vi "AlliGator Load Extended PTU File Information.vi"(8 "Error In":errorcluster, 11 "File Path":path) -> (0 "Error Out":errorcluster, 1 "Data Description":string, 2 "Version":string, 3 "FLI Data File Information":T15, 4 "Load Time (s)":dbl, 5 "Extended ptu File Information":T1, 6 "Magic":string)   [LabVIEW 2021, in "AlliGator Files.lvlib"]
doc: "Extracts metadata used to load FLI dataset from .ptu file."
uses:
  AlliGator Files.lvlib
  AlliGator FLI Data File Information.ctl
  Phasor/Phasor Fluorescence Lifetime Parameters v3.ctl
  AlliGator FLI Dataset Type.ctl
  PicoQuant/PTU/LabVIEW/Extended PicoQuant Data File Information.ctl
  PicoQuant/PTU/LabVIEW/PicoQuant Data File Information.ctl
  PicoQuant/PTU/LabVIEW/PicoQuant File Information.ctl
  PicoQuant/PTU/LabVIEW/PicoQuant Software Information.ctl
  PicoQuant/PTU/LabVIEW/PicoQuant Remote Request Information.ctl
  PicoQuant/PTU/LabVIEW/PicoQuant Hardware Information.ctl
  PicoQuant/PTU/LabVIEW/PicoQuant Input Channels.ctl
  PicoQuant/PTU/LabVIEW/PicoQuant Markers.ctl
  PicoQuant/PTU/LabVIEW/PicoQuant Modules.ctl
  PicoQuant/PTU/LabVIEW/PicoQuant Router Channels.ctl
  PicoQuant/PTU/LabVIEW/PicoQuant Measurement Information.ctl
  PicoQuant/PTU/LabVIEW/PicoQuant Image Information.ctl
  PicoQuant/PTU/LabVIEW/PicoQuant Results Format.ctl
  PicoQuant/PTU/LabVIEW/PicoQuant Measurement Results.ctl
  AlliGator Settings List.ctl
  Variant/Variant to Data/Variant to U32.vi
  AlliGator Load Single Gate Image from PTU File.vi
  PicoQuant/PTU/LabVIEW/PTU Files.lvlib
  PicoQuant/PicoQuant.lvlib
  AlliGator HDF5.lvlib
  AlliGator Settings.lvlib
  Variant/Variant to Data/Variant to Data.lvlib
  Phasor/Phasor.lvlib
panel:
  # "see the AlliGator License on the block diagram (Ctrl+E or Window:Show Block Diagram)"
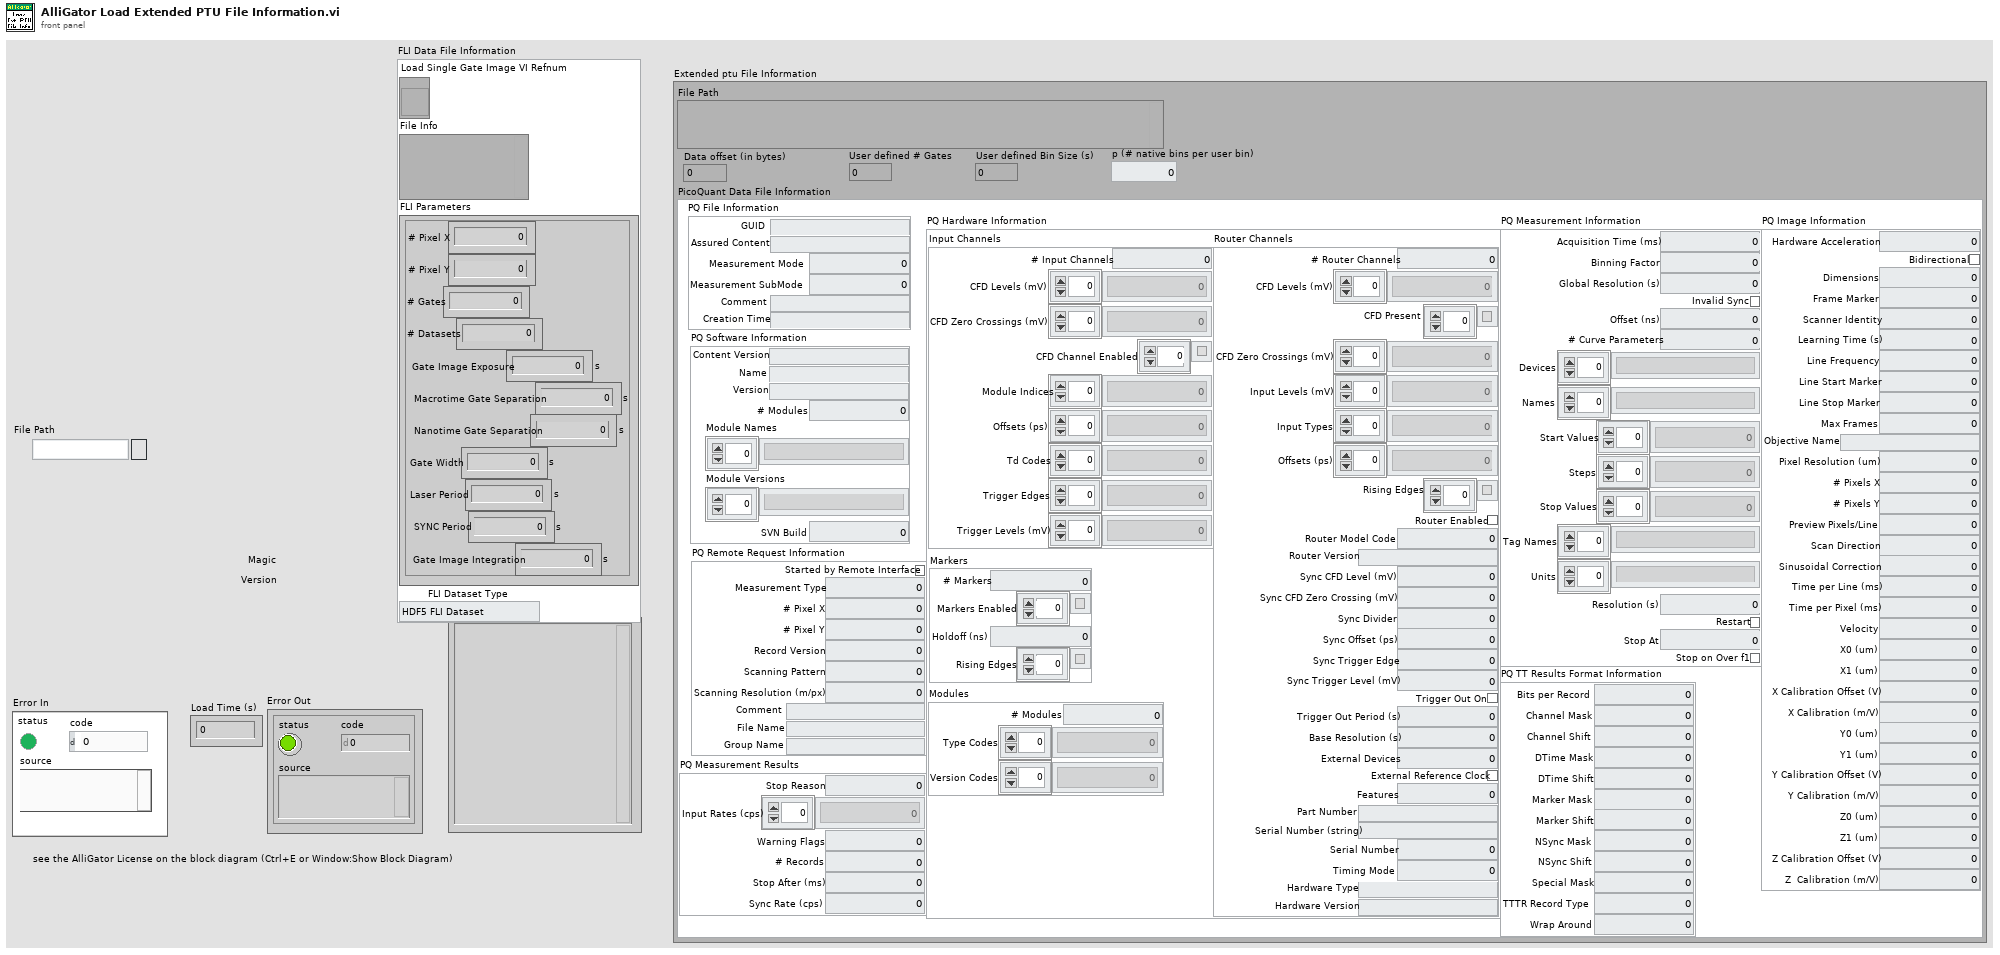
[diagram p1: front panel]
types:
  T1 = typedef "PicoQuant.lvlib/Extended PicoQuant Data File Information.ctl" = cluster{"File Path":path, "Data offset (in bytes)":i64, "PicoQuant Data File Information":T2, "User defined # Gates":i64, "User defined Bin Size (s)":dbl, "p (# native bins per user bin)":dbl}
  T2 = typedef "PTU Files.lvlib/PicoQuant Data File Information.ctl" = cluster{"PQ File Information":T3, "PQ Software Information":T4, "PQ Remote Request Information":T5, "PQ Hardware Information":T6, "PQ Measurement Information":T11, "PQ Image Information":T12, "PQ TT Results Format Information":T13, "PQ Measurement Results":T14}
  T3 = typedef "PTU Files.lvlib/PicoQuant File Information.ctl" = cluster{"GUID":string, "Assured Content":string, "Measurement Mode":i64, "Measurement SubMode":i64, "Comment":string, "Creation Time":string}
  T4 = typedef "PTU Files.lvlib/PicoQuant Software Information.ctl" = cluster{"Content Version":string, "Name":string, "Version":string, "# Modules":i64, "Module Names":string[], "Module Versions":string[], "SVN Build":i64}
  T5 = typedef "PTU Files.lvlib/PicoQuant Remote Request Information.ctl" = cluster{"Started by Remote Interface":bool, "Measurement Type":i64, "# Pixel X":i64, "# Pixel Y":i64, "Record Version":i64, "Scanning Pattern":i64, "Scanning Resolution (m/px)":dbl, "Comment":string, "File Name":string, "Group Name":string}
  T6 = typedef "PTU Files.lvlib/PicoQuant Hardware Information.ctl" = cluster{"Input Channels":T7, "Markers":T8, "Modules":T9, "Router Channels":T10}
  T7 = typedef "PTU Files.lvlib/PicoQuant Input Channels.ctl" = cluster{"# Input Channels":i64, "CFD Levels (mV)":i64[], "CFD Zero Crossings (mV)":i64[], "CFD Channel Enabled":bool[], "Module Indices":i64[], "Offsets (ps)":i64[], "Td Codes":i64[], "Trigger Edges":i64[], "Trigger Levels (mV)":i64[]}
  T8 = typedef "PTU Files.lvlib/PicoQuant Markers.ctl" = cluster{"# Markers":i64, "Markers Enabled":bool[], "Holdoff (ns)":i64, "Rising Edges":bool[]}
  T9 = typedef "PTU Files.lvlib/PicoQuant Modules.ctl" = cluster{"# Modules":i64, "Type Codes":i64[], "Version Codes":i64[]}
  T10 = typedef "PTU Files.lvlib/PicoQuant Router Channels.ctl" = cluster{"# Router Channels":i64, "CFD Levels (mV)":i64[], "CFD Present":bool[], "CFD Zero Crossings (mV)":i64[], "Input Levels (mV)":i64[], "Input Types":i64[], "Offsets (ps)":i64[], "Rising Edges":bool[], "Router Enabled":bool, "Router Model Code":i64, "Router Version":string, "Sync CFD Level (mV)":i64, "Sync CFD Zero Crossing (mV)":i64, "Sync Divider":i64, "Sync Offset (ps)":i64, "Sync Trigger Edge":i64, "Sync Trigger Level (mV)":i64, "Trigger Out On":bool, "Trigger Out Period (s)":dbl, "Base Resolution (s)":dbl, "External Devices":i64, "External Reference Clock":bool, "Features":u64, "Part Number":string, "Serial Number (string)":string, "Serial Number":i64, "Timing Mode":i64, "Hardware Type":string, "Hardware Version":string}
  T11 = typedef "PTU Files.lvlib/PicoQuant Measurement Information.ctl" = cluster{"Acquisition Time (ms)":i64, "Binning Factor":i64, "Global Resolution (s)":dbl, "Invalid Sync":bool, "Offset (ns)":u64, "# Curve Parameters":u64, "Devices":string[], "Names":string[], "Start Values":dbl[], "Steps":dbl[], "Stop Values":dbl[], "Tag Names":string[], "Units":string[], "Resolution (s)":dbl, "Restart":bool, "Stop At":u64, "Stop on Over f1":bool}
  T12 = typedef "PTU Files.lvlib/PicoQuant Image Information.ctl" = cluster{"Hardware Acceleration":i64, "Bidirectional":bool, "Dimensions":i64, "Frame Marker":i64, "Scanner Identity":i64, "Learning Time (s)":i64, "Line Frequency":dbl, "Line Start Marker":i64, "Line Stop Marker":i64, "Max Frames":i64, "Objective Name":string, "Pixel Resolution (um)":dbl, "# Pixels X":i64, "# Pixels Y":i64, "Preview Pixels/Line":i64, "Scan Direction":i64, "Sinusoidal Correction":i64, "Time per Line (ms)":dbl, "Time per Pixel (ms)":i64, "Velocity":i64, "X0 (um)":dbl, "X1 (um)":dbl, "X Calibration Offset (V)":dbl, "X Calibration (m/V)":dbl, "Y0 (um)":dbl, "Y1 (um)":dbl, "Y Calibration Offset (V)":dbl, "Y Calibration (m/V)":dbl, "Z0 (um)":dbl, "Z1 (um)":dbl, "Z Calibration Offset (V)":dbl, "Z  Calibration (m/V)":dbl}
  T13 = typedef "PTU Files.lvlib/PicoQuant Results Format.ctl" = cluster{"Bits per Record":i64, "Channel Mask":i64, "Channel Shift ":i64, "DTime Mask":i64, "DTime Shift":i64, "Marker Mask":i64, "Marker Shift":i64, "NSync Mask":i64, "NSync Shift":i64, "Special Mask":i64, "TTTR Record Type":i64, "Wrap Around":i64}
  T14 = typedef "PTU Files.lvlib/PicoQuant Measurement Results.ctl" = cluster{"Stop Reason":i64, "Input Rates (cps)":i64[], "Warning Flags":u64, "# Records":i64, "Stop After (ms)":i64, "Sync Rate (cps)":i64}
  T15 = typedef "AlliGator HDF5.lvlib/AlliGator FLI Data File Information.ctl" = cluster{"Load Single Gate Image VI Refnum":refnum<vi>, "File Info":variant, "FLI Parameters":T16, "FLI Dataset Type":T17}
  T16 = typedef "Phasor.lvlib/Phasor Fluorescence Lifetime Parameters v3.ctl" = cluster{"# Pixel X":i32, "# Pixel Y":i32, "# Gates":i32, "# Datasets":i32, "Gate Image Exposure":dbl[unit], "Macrotime Gate Separation":dbl[unit], "Nanotime Gate Separation":dbl[unit], "Gate Width":dbl[unit], "Laser Period":dbl[unit], "SYNC Period":dbl[unit], "Gate Image Integration":dbl[unit]}
  T17 = typedef "AlliGator Files.lvlib/AlliGator FLI Dataset Type.ctl" = enum16{"HDF5 FLI Dataset", "Gate Image Folder", ".sdt FLI Dataset (Becker & Hickl)", ".ptu FLI Dataset (PicoQuant)", "SS1 FLI Dataset", "SS2 FLI Dataset", "I/m/phi Dataset", ".bin FLI Dataset (PicoQuant Binned)", ".bin FLI Dataset (Piccolo Binned)"}
  T18 = typedef "AlliGator Settings.lvlib/AlliGator Settings List.ctl" = enum16{"GUI:Visible Settings Tab", "GUI:Last Run Version", "Source Image:Use Image Histogram for Contrast", "Source Image:Low Count Pixels Rejection Options", "Source Image:High Count Pixels Rejection Options", "Source Image:Use Image Brightness", "Source Image:Blend Overlay with Image Background", "Source Image:Use Fixed ROI Diameter", "Source Image:ROI Diameter", "Source Image:ROI Center Color", "Source Image:Peak Threshold", "Source Image:Intensity Threshold", "Source Image:Image Binning Options", "Source Image:Image Smoothing Options", "Source Image:Image Histogram Active", "Source Image:Invert Binary Mask", "Source Image:Hot Pixel Removal", "Source Image:Overlay Analyzed ROI Center", "Source Image:Auto-Adjust Contrast", "Source Image:Histogram Lower Percentile", "Source Image:Histogram Upper Percentile", "Source Image:Save Source Image", "Source Image:Scale Bar Options", "Source Image:Image Resolution (Pixel Size)", "Source Image:Flatfield Correction", "Source Image:Show Dead Left Columns Correction", "Source Image:Dead Left Columns Correction", "Source Image:Image Pre-Processing Operations Order", "Source Image:Overlay ROI Median", "Source Image:Median Overlay Color", "Data Information:Gate Width", "Data Information:Nanotime Gate Separation", "Data Information:Macrotime Gate Separation", "Data Information:Gate Step", "Data Information:# Gates", "Data Information:Gate Image Exposure", "Data Information:Gate Image Integration", "Data Information:Gates to Skip", "Data Information:Gates to Keep", "Data Information:Define Gates to", "Data Information:Channel Name", "Data Information:Available Channel Names", "Data Information:Channel Arithmetic", "Data Information:Background File Subtraction", "Data Information:Background File", "Data Information:Background Scaling Factor", "Data Information:Background Pile-up Correction", "Data Information:Background Pixel Well Capacity", "Data Information:Laser Period", "Data Information:SYNC Period", "Data Information:Pile-up Correction", "Data Information:Pixel Well Capacity", "Data Information:Dataset Scaling Factor", "Fluorescence Decay_Decay Pre-Processing:Reverse Gates", "Fluorescence Decay_Decay Pre-Processing:Verbose Decay Pre-Processing", "Fluorescence Decay_Decay Pre-Processing:Use Decay Pre-Processing", "Fluorescence Decay_Decay Pre-Processing:Background Subtraction", "Fluorescence Decay_Decay Pre-Processing:Background Definition Range", "Fluorescence Decay_Decay Pre-Processing:Baseline Subtraction Method", "Fluorescence Decay_Decay Pre-Processing:Decay Pre-Processing Operations Order", "Fluorescence Decay_Decay Pre-Processing:Smoothing Parameter", "Fluorescence Decay_Decay Pre-Processing:Shift Decay", "Fluorescence Decay_Decay Pre-Processing:Decay Shift Parameters", "Fluorescence Decay_Decay Pre-Processing:Fold Decay", "Fluorescence Decay_Decay Pre-Processing:# Folds", "Fluorescence Decay_Decay Pre-Processing:1-Normalize Decay", "Fluorescence Decay_Decay Pre-Processing:[0-1]-Normalize Decay", "Fluorescence Decay_Decay Pre-Processing:Smoothen Decay", "Fluorescence Decay_Decay Pre-Processing:Extrapolate Decay", "Fluorescence Decay_Decay Pre-Processing:Use Periodicity", "Fluorescence Decay_Decay Pre-Processing:Use Cursors", "Fluorescence Decay_Decay Pre-Processing:Tail Fraction", "Fluorescence Decay_Decay Pre-Processing:Head Fraction", "Fluorescence Decay_Decay Pre-Processing:Additional Points", "Fluorescence Decay_Decay Pre-Processing:Straighten Decay", "Fluorescence Decay_Decay Pre-Processing:Constant Background", "Fluorescence Decay_Decay Pre-Processing:Pixel-Normalize Decay", "Fluorescence Decay_Advanced Analysis:Extract IRF instead of Decay", "Fluorescence Decay_Advanced Analysis:IRF Extraction Options", "Fluorescence Decay_Advanced Analysis:IRF Optimization Options", "Fluorescence Decay_Advanced Analysis:Square Pulse Options", "Fluorescence Decay_Advanced Analysis:IRF Order", "Fluorescence Decay_Advanced Analysis:IRF Time Constants", "Fluorescence Decay_Advanced Analysis:Wavelet Analysis Options", "Fluorescence Decay_Advanced Analysis:Average Lifetime Options", "Fluorescence Decay_Fit Options:Fit Options", "Fluorescence Decay_Fit Options:Use Legacy Fitting Approach", "Fluorescence Decay_Fit Options:Use Data Information Laser Period", "Fluorescence Decay_Fit Parameters:Displayed Fit Parameters", "Fluorescence Decay_Fit Parameters:Fit Parameter Constraints", "Fluorescence Decay_Fit Parameters:Export Tabulated Results", "Fluorescence Decay_Fit Parameters:MLE Baseline Offset Type", "Fluorescence Decay_Fit Parameters:MLE Baseline Offset", "Fluorescence Decay_Fit Parameters:Guess Parameter Names", "Fluorescence Decay_Fit Parameters:Guess Parameter Values", "Fluorescence Decay_Fit Parameters:Guess Parameters Options", "Fluorescence Decay_Styles:Show Last Decay Only", "Fluorescence Decay_Styles:Decay Graph Color Array", "Fluorescence Decay:Decay Graph Active", "Fluorescence Decay Statistics:Min Peak Value", "Fluorescence Decay Statistics:Reject Low Decay Peak Pixels", "Fluorescence Decay Statistics:Reject High Decay Peak Pixels", "Fluorescence Decay Statistics:Max Peak Value", "Time Traces:Use File Timestamp", "Time Traces:Time Step", "Time Traces:Use Intensity Correction File", "Time Traces:Intensity Correction File", "Phasor Plot:Phasor Plot Smoothing Options", "Phasor Plot:Phasor Plot Size", "Phasor Plot:Phasor Plot Graphics Options", "Phasor Plot:Cumulative Phasor Plot", "Phasor Plot:Use Phasor Brightness", "Phasor Plot:Blend Overlay with Phasor Background", "Phasor Plot:Save Phasor Plot", "Phasor Plot:Show References", "Phasor Plot:Phasor Ratio Decay Range", "Phasor Plot:Exponential Fading", "Phasor Plot:Phasor Ratio Reference Colors", "Phasor Plot:Reference Radius", "Phasor Plot:Show Color Map Vertices", "Phasor Plot:Phasor Plot Active", "Phasor Plot:Phasor Ratio Color Map Type", "Phasor Plot:Phasor Ratio Color Map", "Phasor Plot:Phasor Ratio Display Range", "Phasor Plot:Selected Image ROI(s)", "Phasor Plot:All Image ROIs", "Phasor Plot:Selected Phasor Plot ROI(s)", "Phasor Plot:All Phasor Plot ROIs", "Phasor Plot:Phasor Ratio Color-Coded Quantity", "Phasor Plot:Store Phasor Harmonics", "Phasor Plot:Draw Reference Segment", "Phasor Plot:User-Defined Quantity", "Phasor Graph:Phasor Frequency", "Phasor Graph:Phasor Ratio Type", "Phasor Graph:Pixel-level Phasor Computation", "Phasor Graph:Save Phasor Graph", "Phasor Graph:Phasor Graph Active", "Phasor Graph:Phasor SDV Options", "Phasor Calibration:Use Backup Calibration if needed", "Phasor Graph:Define Shortest Lifetime as", "Phasor Calibration:Backup Calibration Type", "Phasor Calibration:Calibration Type", "Phasor Calibration:Calibration Lifetime", "Phasor Calibration:Calibration Map Algorithm", "Single-Exponential Phasor Locus (SEPL):Gate Parameters", "Single-Exponential Phasor Locus (SEPL):User-defined Gate", "Single-Exponential Phasor Locus (SEPL):User-defined IRF", "Single-Exponential Phasor Locus (SEPL):Phasor Parameters", "Single-Exponential Phasor Locus (SEPL):Decay & IRF Parameters", "Single-Exponential Phasor Locus (SEPL):Display Parameters", "Lifetime Analysis:Decay Analysis Parameters", "Lifetime Analysis:Lifetime Map Active", "Plugins:Python Settings", "Miscellaneous:Verbose Mode", "Miscellaneous:Beep after Script", "Miscellaneous:Saved Image File Format", "Miscellaneous:Exported Gate Image Settings", "Miscellaneous:Include Loading in Timing", "Miscellaneous:Verbose Settings Mode", "Miscellaneous:Histogram Options", "Miscellaneous:Beep on Error", "Miscellaneous:# Logical Processors Used", "Miscellaneous:ROI Description Max Characters", "Miscellaneous:Verbose Error Mode", "Miscellaneous:Transparent Mask Color"}
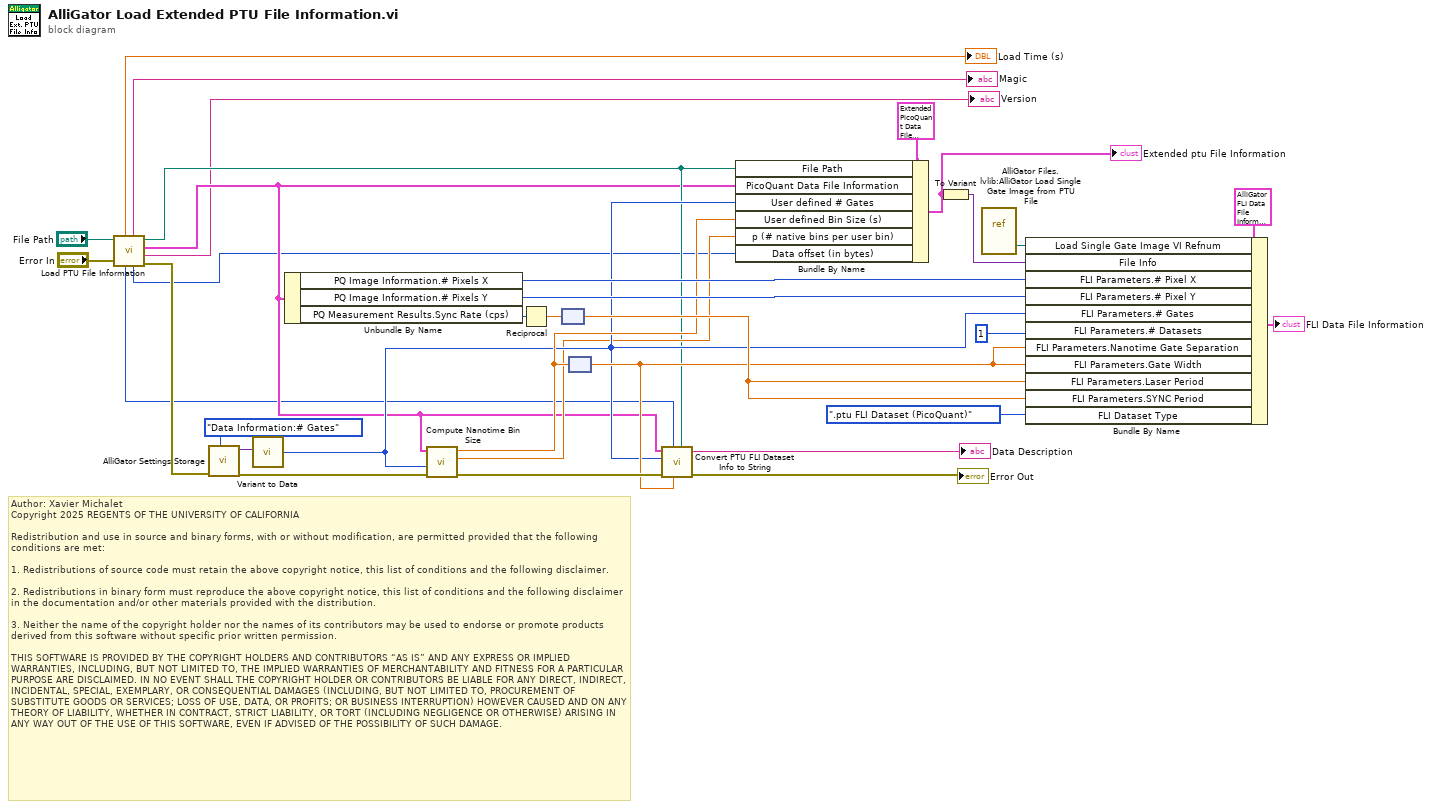
[diagram p0: block diagram]
diagram:
  # "Author: Xavier Michalet\nCopyright 2025 REGENTS OF THE UNIVERSITY OF CALIFORNIA\n\nRedistribution and use in source and binary forms, with or without modification, are permitted provided that the following conditions are met:\n\n1. Redistributions of source code must retain the above copyright notice, this list of conditions and the following disclaimer.\n\n2. Redistributions in binary form must reproduce the above copyright notice, this list of conditions and the following disclaimer in the documentation and/or other materials provided with the distribution.\n\n3. Neither the name of the copyright holder nor the names of its contributors may be used to endorse or promote products derived from this software without specific prior written permission.\n\nTHIS SOFTWARE IS PROVIDED BY THE COPYRIGHT HOLDERS AND CONTRIBUTORS “AS IS” AND ANY EXPRESS OR IMPLIED WARRANTIES, INCLUDING, BUT NOT LIMITED TO, THE IMPLIED WARRANTIES OF MERCHANTABILITY AND FITNESS FOR A PARTICULAR PURPOSE ARE DISCLAIMED. IN NO EVENT SHALL THE COPYRIGHT HOLDER OR CONTRIBUTORS BE LIABLE FOR ANY DIRECT, INDIRECT, INCIDENTAL, SPECIAL, EXEMPLARY, OR CONSEQUENTIAL DAMAGES (INCLUDING, BUT NOT LIMITED TO, PROCUREMENT OF SUBSTITUTE GOODS OR SERVICES; LOSS OF USE, DATA, OR PROFITS; OR BUSINESS INTERRUPTION) HOWEVER CAUSED AND ON ANY THEORY OF LIABILITY, WHETHER IN CONTRACT, STRICT LIABILITY, OR TORT (INCLUDING NEGLIGENCE OR OTHERWISE) ARISING IN ANY WAY OUT OF THE USE OF THIS SOFTWARE, EVEN IF ADVISED OF THE POSSIBILITY OF SUCH DAMAGE."
  n1 = call "Load PTU File Information.vi"("error in (no error)"="Error In", "File Path"="File Path") -> ("error out"=w8:errorcluster, "Version"=→"Version":string, "PicoQuant Data File Information"=w4:T2, "path (dup)"=w7:path, "Data offset (in bytes)"=w2:i64, "Magic"=→"Magic":string, "size (in bytes)"=w1:i64, "elapsed (relative) seconds"=→"Load Time (s)":dbl)  [unwired: 2 in]
  n2 = call "AlliGator Settings Storage.vi"("AlliGator Settings List"=AlliGator_Settings_List."Data Information:# Gates", "Error In"=w8) -> ("Error Out"=w13:errorcluster, "Variant Data out"=w14:variant)  [unwired: 8 in]
  n3 = call-poly "Variant to Data.vi"("Variant"=w14) -> ("Value"=w11:u32)  [unwired: 8 in]
  n4 = Unbundle By Name(w4) -> ("PQ Image Information.# Pixels X"=w19:i64, "PQ Image Information.# Pixels Y"=w18:i64, "PQ Measurement Results.Sync Rate (cps)"=w30:i64)
  n5 = call "Compute Nanotime Bin Size.vi"("Error In"=w13, "# Gates"=w11, "PicoQuant Data File Information"=w4) -> ("Error Out"=w21:errorcluster, "p (# native bins per user bin)"=w9:dbl, "user bin size (Gate Step & Width) (s)"=w15:dbl)  [unwired: 6 in]
  n6 = Reciprocal(x=w30) -> (1/x=w29:dbl)
  n7 = node(w29) -> (w23:dbl[unit])
  n8 = node(w15) -> (w17:dbl[unit])
  n9 = call "Convert PTU FLI Dataset Info to String.vi"("File Path"=w7, "Step Duration"=w17, "File Size"=w1, "error in (no error)"=w21, "# Frames"=w11, "PTU File Information"=w4) -> ("Error Out"=→"Error Out":errorcluster, "Data Description"=→"Data Description":string)  [unwired: 4 in]
  n10 = Bundle By Name(cluster=T1 {"File Path"=path "", "Data offset (in bytes)"=0, "PicoQuant Data File Information"={"PQ File Information"={"GUID"="", "Assured Content"="", "Measurement Mode"=0, "Measurement SubMode"=0, "Comment"="", "Creation Time"=""}, "PQ Software Information"={"Content Version"="", "Name"="", "Version"="", "# Modules"=0, "Module Names"=[], "Module Versions"=[], "SVN Build"=0}, "PQ Remote Request Information"={"Started by Remote Interface"=FALSE, "Measurement Type"=0, "# Pixel X"=0, "# Pixel Y"=0, "Record Version"=0, "Scanning Pattern"=0, "Scanning Resolution (m/px)"=0.0, "Comment"="", "File Name"="", "Group Name"=""}, "PQ Hardware Information"={"Input Channels"={"# Input Channels"=0, "CFD Levels (mV)"=[], "CFD Zero Crossings (mV)"=[], "CFD Channel Enabled"=[], "Module Indices"=[], "Offsets (ps)"=[], "Td Codes"=[], "Trigger Edges"=[], "Trigger Levels (mV)"=[]}, "Markers"={"# Markers"=0, "Markers Enabled"=[], "Holdoff (ns)"=0, "Rising Edges"=[]}, "Modules"={"# Modules"=0, "Type Codes"=[], "Version Codes"=[]}, "Router Channels"={"# Router Channels"=0, "CFD Levels (mV)"=[], "CFD Present"=[], "CFD Zero Crossings (mV)"=[], "Input Levels (mV)"=[], "Input Types"=[], "Offsets (ps)"=[], "Rising Edges"=[], "Router Enabled"=FALSE, "Router Model Code"=0, "Router Version"="", "Sync CFD Level (mV)"=0, "Sync CFD Zero Crossing (mV)"=0, "Sync Divider"=0, "Sync Offset (ps)"=0, "Sync Trigger Edge"=0, "Sync Trigger Level (mV)"=0, "Trigger Out On"=FALSE, "Trigger Out Period (s)"=0.0, "Base Resolution (s)"=0.0, "External Devices"=0, "External Reference Clock"=FALSE, "Features"=0, "Part Number"="", "Serial Number (string)"="", "Serial Number"=0, "Timing Mode"=0, "Hardware Type"="", "Hardware Version"=""}}, "PQ Measurement Information"={"Acquisition Time (ms)"=0, "Binning Factor"=0, "Global Resolution (s)"=0.0, "Invalid Sync"=FALSE, "Offset (ns)"=0, "# Curve Parameters"=0, "Devices"=[], "Names"=[], "Start Values"=[], "Steps"=[], "Stop Values"=[], "Tag Names"=[], "Units"=[], "Resolution (s)"=0.0, "Restart"=FALSE, "Stop At"=0, "Stop on Over f1"=FALSE}, "PQ Image Information"={"Hardware Acceleration"=0, "Bidirectional"=FALSE, "Dimensions"=0, "Frame Marker"=0, "Scanner Identity"=0, "Learning Time (s)"=0, "Line Frequency"=0.0, "Line Start Marker"=0, "Line Stop Marker"=0, "Max Frames"=0, "Objective Name"="", "Pixel Resolution (um)"=0.0, "# Pixels X"=0, "# Pixels Y"=0, "Preview Pixels/Line"=0, "Scan Direction"=0, "Sinusoidal Correction"=0, "Time per Line (ms)"=0.0, "Time per Pixel (ms)"=0, "Velocity"=0, "X0 (um)"=0.0, "X1 (um)"=0.0, "X Calibration Offset (V)"=0.0, "X Calibration (m/V)"=0.0, "Y0 (um)"=0.0, "Y1 (um)"=0.0, "Y Calibration Offset (V)"=0.0, "Y Calibration (m/V)"=0.0, "Z0 (um)"=0.0, "Z1 (um)"=0.0, "Z Calibration Offset (V)"=0.0, "Z  Calibration (m/V)"=0.0}, "PQ TT Results Format Information"={"Bits per Record"=0, "Channel Mask"=0, "Channel Shift "=0, "DTime Mask"=0, "DTime Shift"=0, "Marker Mask"=0, "Marker Shift"=0, "NSync Mask"=0, "NSync Shift"=0, "Special Mask"=0, "TTTR Record Type"=0, "Wrap Around"=0}, "PQ Measurement Results"={"Stop Reason"=0, "Input Rates (cps)"=[], "Warning Flags"=0, "# Records"=0, "Stop After (ms)"=0, "Sync Rate (cps)"=0}}, "User defined # Gates"=0, "User defined Bin Size (s)"=0.0, "p (# native bins per user bin)"=0.0} ("Extended PicoQuant Data File Information"), "File Path"=w7, "PicoQuant Data File Information"=w4, "User defined # Gates"=w11, "User defined Bin Size (s)"=w15, "p (# native bins per user bin)"=w9, "Data offset (in bytes)"=w2) -> (w26:T1)
  "Extended ptu File Information" <- w26
  n11 = To Variant(anything=w26) -> (Variant=w25:variant)
  n12 = vi-ref "AlliGator Files.lvlib:AlliGator Load Single Gate Image from PTU File.vi"() -> (w16:refnum<vi>)
  n13 = Bundle By Name(cluster=T15 {"Load Single Gate Image VI Refnum"=refnum, "File Info"=variant, "FLI Parameters"={"# Pixel X"=0, "# Pixel Y"=0, "# Gates"=0, "# Datasets"=0, "Gate Image Exposure"=0.0, "Macrotime Gate Separation"=0.0, "Nanotime Gate Separation"=0.0, "Gate Width"=0.0, "Laser Period"=0.0, "SYNC Period"=0.0, "Gate Image Integration"=0.0}, "FLI Dataset Type"=enum."HDF5 FLI Dataset"} ("FLI Data File Information"), "Load Single Gate Image VI Refnum"=w16, "File Info"=w25, "FLI Parameters.# Pixel X"=w19, "FLI Parameters.# Pixel Y"=w18, "FLI Parameters.# Gates"=w11, "FLI Parameters.# Datasets"=1, "FLI Parameters.Nanotime Gate Separation"=w17, "FLI Parameters.Gate Width"=w17, "FLI Parameters.Laser Period"=w23, "FLI Parameters.SYNC Period"=w23, "FLI Dataset Type"=AlliGator_FLI_Dataset_Type.".ptu FLI Dataset (PicoQuant)") -> (→"FLI Data File Information":T15)
